vi "Mensaje falta dinero.vi"(10 "Msj":enum16{"ESP", "ING"}(ring), 11 "Message Enqueuer in":refnum<class "Message Enqueuer.lvclass">) -> ()   [LabVIEW 2019, in "UI Actor.lvlib" / "UI Actor.lvclass"]
uses:
  UI Actor.lvclass
  <vilib>/ActorFramework/Message Enqueuer/Message Enqueuer.lvclass
  Mensajes Actor Messages/Update Msj Msg/Update Msj Msg.lvclass/Update Msj Msg.ctl
  <vilib>/ActorFramework/Message Enqueuer/Message Enqueuer.lvclass/Message Enqueuer.ctl
  <vilib>/ActorFramework/Message Enqueuer/Enqueue.vi
  Mensajes Actor Messages/Update Msj Msg/Update Msj Msg.lvclass
  C:/Program Files/National Instruments/LabVIEW 2019/vi.lib/ActorFramework/Message/Message.lvclass
  <vilib>/ActorFramework/Message Priority Queue/Priority Enqueue.vi
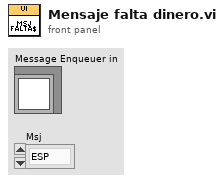
[diagram p1: front panel]
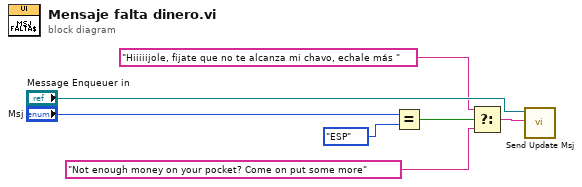
[diagram p0: block diagram]
diagram:
  n1 = Equal?(x="Msj", y=enum16{"ESP", "ING"}."ESP") -> (x = y?=w1:bool)
  n2 = Select(t="Hiiiiijole, fijate que no te alcanza mi chavo, echale más ", s=w1, f="Not enough money on your pocket? Come on put some more") -> (s? t:f=w2:string)
  n3 = call "Send Update Msj.vi"("Update Msj"=w2, "Message Enqueuer"="Message Enqueuer in") -> ()  [unwired: 8 in, 2 out]
